vi "Init Attributes.vi"(10 "Attributes":T1) -> (3 "Base Attributes out":refnum<class "Base Attributes.lvclass">)   [LabVIEW 2020, in "jettl.lvlib" / "Base Attributes.lvlib" / "Base Attributes.lvclass"]
uses:
  Base Attributes.lvclass
  Attributes.ctl
  Attributes/Attributes.lvclass
  Transport/Transport.lvclass
  Msgs.ctl
  Msg/Msg.lvclass
  Actor/Actor.lvclass
  Base Attributes.lvclass/Base Attributes.ctl
  jettl.lvlib
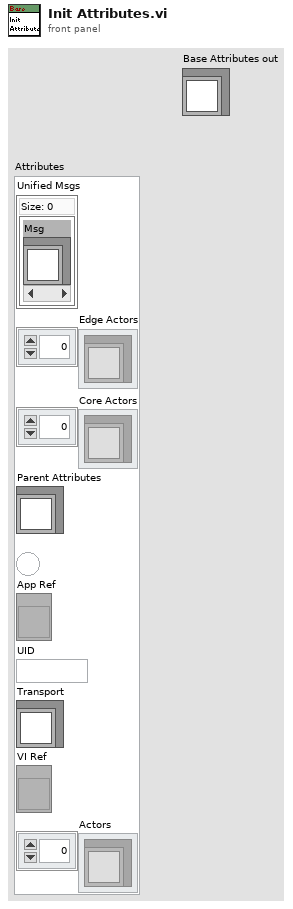
[diagram p1: front panel]
types:
  T1 = typedef "jettl.lvlib/Attributes.ctl" = cluster{"Unified Msgs":T2, "Edge Actors":refnum<class "Actor.lvclass">[], "Core Actors":refnum<class "Actor.lvclass">[], "Parent Attributes":refnum<class "Attributes.lvclass">, "Root":bool, "App Ref":refnum<vi>, "UID":string, "Transport":refnum<class "Transport.lvclass">, "VI Ref":refnum<vi>, "Actors":refnum<class "Actor.lvclass">[]}
  T2 = typedef "jettl.lvlib/Msgs.ctl" = set{refnum<class "Msg.lvclass">}
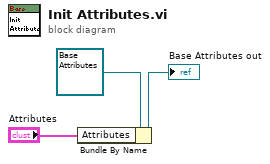
[diagram p0: block diagram]
diagram:
  n1 = Bundle By Name(cluster=refnum<class "Base Attributes.lvclass"> refnum ("Base Attributes in"), "Attributes"="Attributes") -> (→"Base Attributes out":refnum<class "Base Attributes.lvclass">)
